vi "Do.vi"(8 "error in (no error)":errorcluster, 10 "Actor in":refnum<class "Actor.lvclass">, 11 "Update DemoService Msg":refnum<class "Update DemoService Msg.lvclass">) -> (0 "error out":errorcluster, 2 "Actor out":refnum<class "Actor.lvclass">)   [LabVIEW 2012, in "DimActorDemo.lvlib" / "Update DemoService Msg.lvclass"]
doc: "This VI delivers the message to the actor by calling the appropriate method(s) on the actor."
uses:
  Update DemoService Msg.lvclass
  <vilib>/ActorFramework/Actor/Actor.lvclass
  DIMDemoServer/DIMDemoServer.lvclass
  Update DemoService Msg.lvclass/Update DemoService Msg.ctl
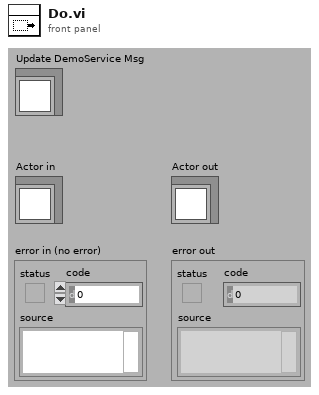
[diagram p1: front panel]
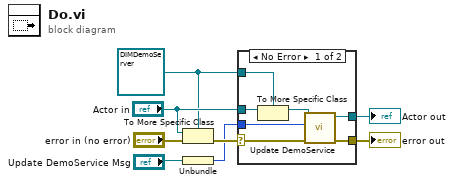
[diagram p0: block diagram]
diagram:
  w2 = refnum<class "DIMDemoServer.lvclass"> refnum ("Actor in")
  n1 = To More Specific Class(target class=w2, reference="Actor in", error in="error in (no error)") -> (error out=w6:errorcluster)  [unwired: 1 out]
  n2 = Unbundle("Update DemoService Msg") -> (w1:i32)
  n3 = case shown="No Error" w6 {
    selector: w6 -> [w13 w17]
    tunnel: [w15 w17] -> w5
    tunnel: [w14 w16] -> w4
    tunnel: "Actor in" -> [w12 w16]
    tunnel: w2 -> [w11 _]
    tunnel: w1 -> [w9 _]
    frame No Error {
      n4 = To More Specific Class(target class=w11, reference=w12) -> (specific class reference=w10:refnum<class "DIMDemoServer.lvclass">)  [unwired: 1 in, 1 out]
      n5 = call "Update DemoService.vi"("error in (no error)"=w13, "DemoService"=w9, "DIMDemoServer in"=w10) -> ("error out"=w15:errorcluster, "DIMDemoServer out"=w14:refnum<class "DIMDemoServer.lvclass">)  [unwired: 7 in]
    }
    frame Error {
    }
  }
  "error out" <- w5
  "Actor out" <- w4
